vi "Set_Radio_Device_Name.vi"(8 "error in (no error)":errorcluster, 9 "value":string(combo)="0", 10 "Cellular Technology":T1, 11 "Base Station":T2) -> (0 "error out":errorcluster, 3 "Output String":string)   [LabVIEW 2021]
uses:
  Controls/Base_Station_Emulator.ctl
  Controls/Cellular_Technology.ctl
  Controls/TCP_FGV.ctl
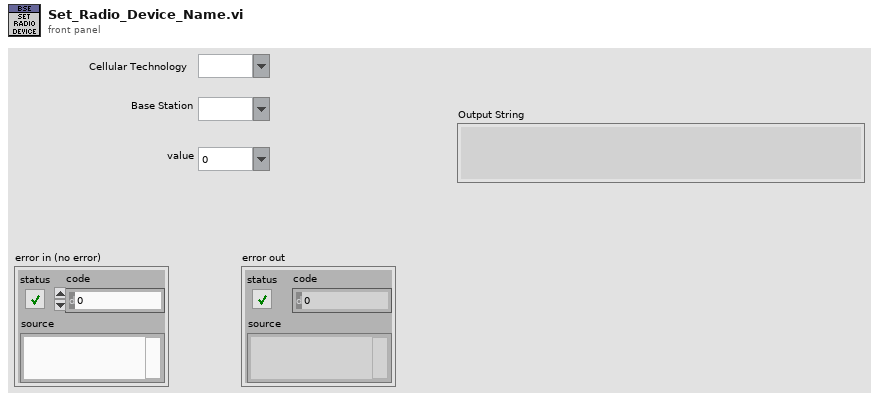
[diagram p1: front panel]
types:
  T1 = typedef "Cellular_Technology.ctl" = string
  T2 = typedef "Base_Station_Emulator.ctl" = string
  T3 = typedef "TCP_FGV.ctl" = enum16{"Open", "Read", "Write", "Close"}
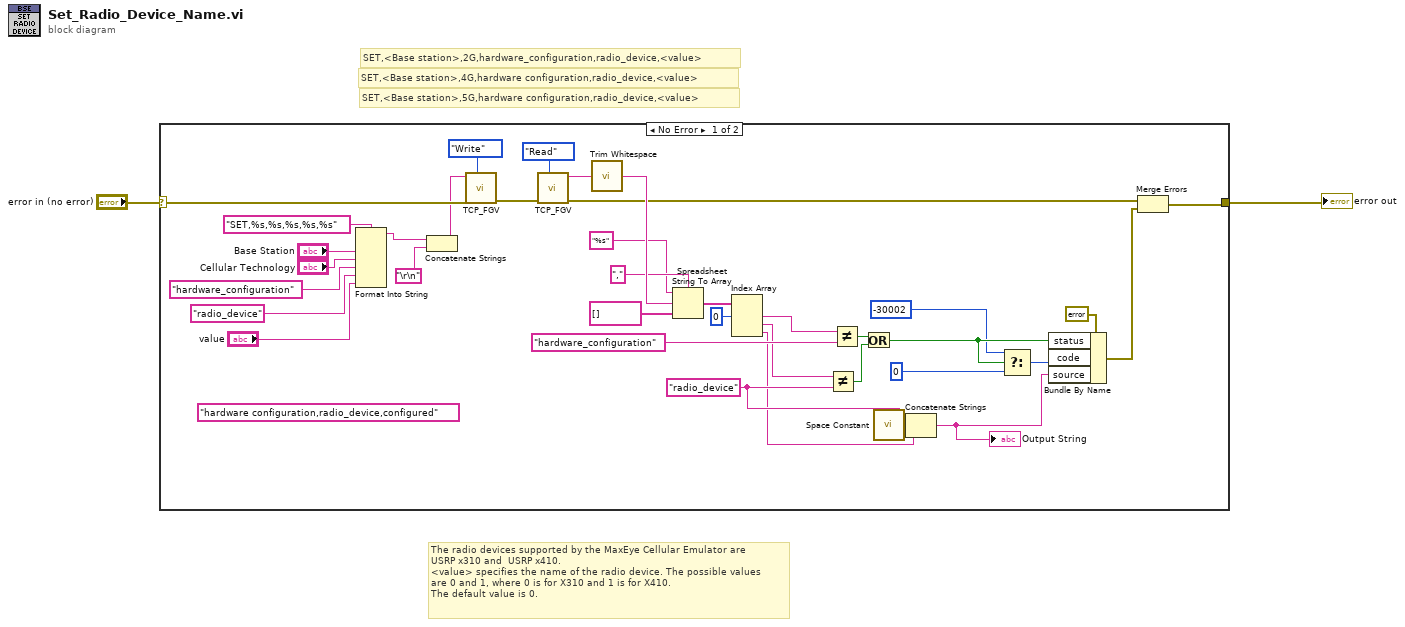
[diagram p0: block diagram]
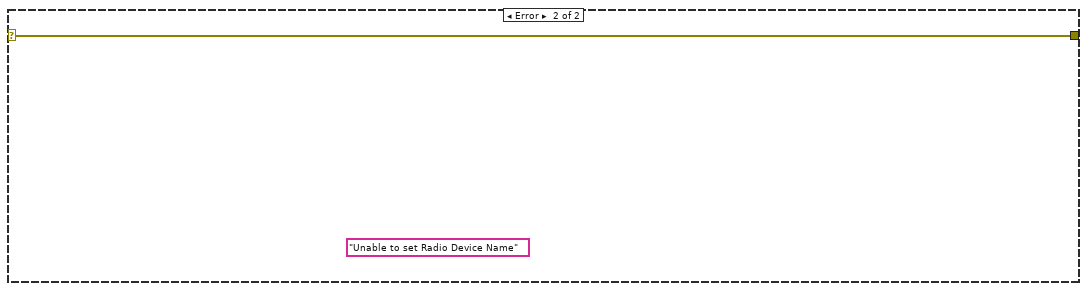
[diagram p2: hidden frame]
diagram:
  # "The radio devices supported by the MaxEye Cellular Emulator are   \nUSRP x310 and  USRP x410. \n<value> specifies the name of the radio device. The possible values \nare 0 and 1, where 0 is for X310 and 1 is for X410. \nThe default value is 0."
  # "SET,<Base station>,5G,hardware configuration,radio_device,<value>"
  # "SET,<Base station>,4G,hardware configuration,radio_device,<value>"
  # "SET,<Base station>,2G,hardware_configuration,radio_device,<value>"
  n1 = case shown="No Error" "error in (no error)" {
    selector: "error in (no error)" -> [w36 w40]
    tunnel: [w15 w40] -> w2
    frame No Error {
      (unwired) "hardware configuration,radio_device,configured" ("format string")
      w11 = "radio_device"
      n2 = Format Into String(format string="SET,%s,%s,%s,%s,%s", "Base Station", "Cellular Technology", "hardware_configuration", "radio_device", "value") -> (resulting string=w5:string)  [unwired: 2 in, 1 out]
      n3 = Concatenate Strings(w5, "\r\n") -> (w4:string)
      n4 = call "TCP_FGV.vi"("Command"=w4, "error in (no error)"=w36, "Operation"=TCP_FGV."Write") -> ("error out"=w33:errorcluster)  [unwired: 6 in, 1 out]
      n5 = call "TCP_FGV.vi"("error in (no error)"=w33, "Operation"=TCP_FGV."Read") -> ("Data Out"=w13:string, "error out"=w17:errorcluster)  [unwired: 7 in]
      n6 = call <vilib>:"Trim Whitespace.vi"("string"=w13) -> ("trimmed string"=w28:string)  [unwired: 1 in]
      n7 = Spreadsheet String To Array(delimiter (Tab)=",", format string="%s", spreadsheet string=w28, array type (2D Dbl)=string[] []) -> (array=w32:string[])
      n8 = Index Array(array=w32, index #1=0 ("index")) -> (element #1=w31:string, element #2=w14:string, element #3=w10:string)  [unwired: 2 in]
      n9 = Not Equal?(x=w14, y=w11) -> (x != y?=w29:bool)
      n10 = Not Equal?(x=w31, y="hardware_configuration" ("format string")) -> (x != y?=w30:bool)
      n11 = Or(x=w30, y=w29) -> (x .or. y?=w27:bool)
      n12 = call <vilib>:"Space Constant.vi"() -> ("String"=w12:string)
      n13 = Concatenate Strings(w11, w12, w10) -> (w9:string)
      "Output String" <- w9
      n14 = Select(t=-30002 ("code"), s=w27, f=0 ("code")) -> (s? t:f=w26:i32)
      n15 = Bundle By Name(cluster=errorcluster {"status"=FALSE, "code"=0, "source"=""} ("error constant"), "status"=w27, "code"=w26, "source"=w9) -> (w16:errorcluster)
      n16 = Merge Errors(w17, w16) -> (w15:errorcluster)
    }
    frame Error {
      (unwired) "Unable to set Radio Device Name" ("source")
    }
  }
  "error out" <- w2
